vi "GetEvent.vi"(8 "error in":errorcluster) -> (0 "error out":errorcluster, 3 "Event":refnum<user-event>)   [LabVIEW 2012, in "Spinner.xctl"]
uses:
  Spinner.xctl
  EventData.ctl
  Command.ctl
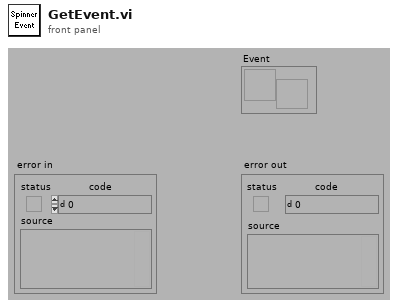
[diagram p1: front panel]
types:
  T1 = typedef "Spinner.xctl/EventData.ctl" = cluster{"Step Len":dbl, "Pic Ref":refnum<vi>, "Ctrl Ref":u32, "Imgs":picture[], "Command":T2}
  T2 = typedef "Spinner.xctl/Command.ctl" = enum16{"Add Control", "Remove Control", "Update Imgs", "Update Speed", "Refresh"}
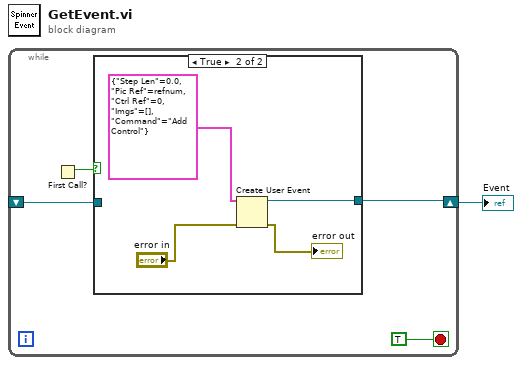
[diagram p0: block diagram]
diagram:
  n1 = while {
    shift-right: [w3] -> w1
    shift-left: _ -> [w2]
    stop <- TRUE stop-if-true
    n2 = First Call?() -> (First Call?: T/F=w4:bool)
    n3 = case shown="True" w4 {
      tunnel: [w6 w10] -> w3
      tunnel: w2 -> [w6 _]
      frame False {
      }
      frame True {
        n4 = Create User Event(user event datatype=T1 {"Step Len"=0.0, "Pic Ref"=refnum, "Ctrl Ref"=0, "Imgs"=[], "Command"=enum."Add Control"} ("Spinner event datatype"), error in="error in") -> (user event=w10:refnum<user-event>, error out=→"error out":errorcluster)
      }
    }
  }
  "Event" <- w1
